vi "pwm test.vi"() -> ()   [LabVIEW 2019, in "my FPGA lib.lvlib" / "motor.lvlib"]
uses:
  motor.lvlib
  <vilib>/Platform/TimedLoop/XDataNode/timing_clust.ctl
  <vilib>/Platform/TimedLoop/XDataNode/nitl_modes.ctl
  <vilib>/Platform/TimedLoop/XDataNode/wakeup.ctl
  motor enum.ctl
  <vilib>/platform/TimedLoop/XDataNode/XDataNode.xnode
  my FPGA lib.lvlib
  <vilib>/Platform/TimedLoop/XDataNode/XDNodeRunTimeDep.lvlib
panel:
  out "error out":errorcluster
  in  "PWM":dbl
  in  "Reset":bool
  in  "Stop":bool
  in  "PWM frequence":dbl
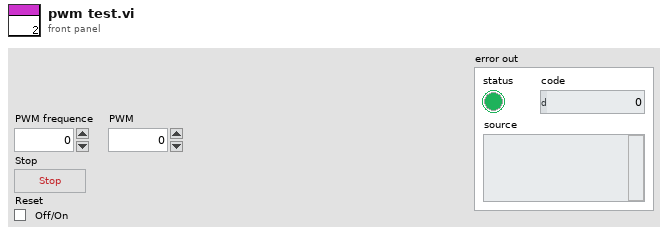
[diagram p1: front panel]
types:
  T1 = typedef "XDNodeRunTimeDep.lvlib/timing_clust.ctl" = cluster{"Expected End [f-1]":u64, "Actual End [f-1]":u64, "Finished Late? [f-1]":bool, "Expected End [i-1]":u64, "Actual End [i-1]":u64, "Finished Late? [i-1]":bool, "Expected Start [i]":u64, "Actual Start [i]":u64, "Expected Start [f]":u64, "Actual Start [f]":u64, "Source Name":string, "Structure Name":string, "Period":i64, "Deadline":i64, "Offset":i64, "Start":i64, "Priority":i32, "Timeout":i32, "Mode":T2, "Wakeup Reason":T3, "Error":errorcluster, "Source Type":string, "Secondary Source Type":string, "Global End Time":u64, "Global Start Time":u64, "Frame Duration":u64, "Iteration Duration":u64, "Assigned CPU":i32, "I/O Scan Engine Mode":u32}
  T2 = typedef "XDNodeRunTimeDep.lvlib/nitl_modes.ctl" = enum32{"No Change", "Process missed periods, maintain original phase", "Discard missed periods, maintain original phase", "Process missed periods, ignore original phase", "Discard missed periods, ignore original phase"}
  T3 = typedef "XDNodeRunTimeDep.lvlib/wakeup.ctl" = enum32{"Normal", "Aborted", "Asynchronous wakeup", "Timing source error", "Timed loop error", "Timeout"}
  T4 = typedef "my FPGA lib.lvlib/motor.lvlib/motor enum.ctl" = enum16{"M1", "M2", "M3", "M4"}
  T5 = cluster{"divider rate":i32, "enable divider":bool, "period":i32}
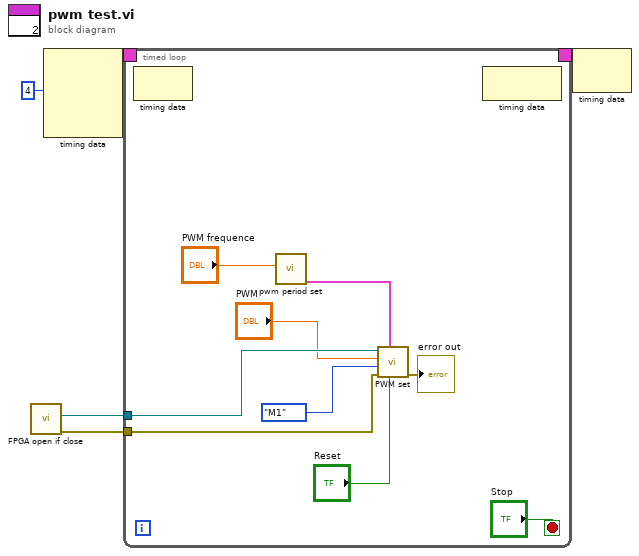
[diagram p0: block diagram]
diagram:
  n1 = call "FPGA open if close.vi"() -> ("error out"=w1:errorcluster, "FPGA VI Reference Out"=w5:refnum<k20>)  [unwired: 10 in]
  n2 = node-c288(i64 4 ("Period")) -> (w4:T1)  [unwired: 3 in]
  n3 = timed-loop {
    timing: w4 -> [_]
    timing-out: [_] -> w3
    tunnel: w5 -> [w13]
    tunnel: w1 -> [w10]
    stop <- "Stop" stop-if-true
    n4 = node-c288() -> ()  [unwired: 1 in, 1 out]
    n5 = call "pwm period set.vi"("PWM frequence"="PWM frequence") -> ("pwm cnfg"=w12:T5)  [unwired: 10 in]
    n6 = call "PWM set.vi"("Reset"="Reset", "pwm cnfg"=w12, "Error In"=w10, "motor select"=motor_enum."M1", "PWM"="PWM", "FPGA VI Reference In"=w13) -> ("error out"=→"error out":errorcluster)  [unwired: 5 in]
    n7 = node-c288() -> ()  [unwired: 1 in, 1 out]
  }
  n8 = node-c288(w3) -> ()  [unwired: 1 out]
